vi "list and create PG DI table_1.vi"(8 "error in":errorcluster, 9 "DI table":string[](array[string]), 10 "table name":string, 11 "conn":u32) -> (0 "error out":errorcluster, 3 "conn_out":u32)   [LabVIEW 2019, in "PostgreSQL.lvlib"]
uses:
  PostgreSQL.lvlib
  PostgreSQL2LabVIEW/libpqlv/src/PQresultErrorMessage.vi
  PostgreSQL2LabVIEW/libpqUtility/src/PQclear.vi
  PostgreSQL2LabVIEW/libpqlv/src/PQsendQuery.vi
  PostgreSQL2LabVIEW/libpqlv/src/PQgetResult.vi
  PostgreSQL2LabVIEW/libpqlv/src/PQresultStatus.vi
  PostgreSQL2LabVIEW/libpqUtility/src/PQgetColumn.vi
  PostgreSQL2LabVIEW/libpqlv/src/PQclear.vi
  PostgreSQL2LabVIEW/libpqUtility/src/PQfetchTables.vi
  PostgreSQL2LabVIEW/libpqlv/src/PQgetvalue.vi
  PostgreSQL2LabVIEW/libpqlv/src/PQntuples.vi
  PostgreSQL2LabVIEW/libpqUtility/libpqutility.lvlib
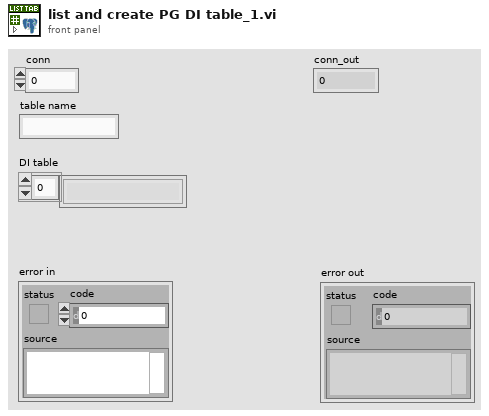
[diagram p1: front panel]
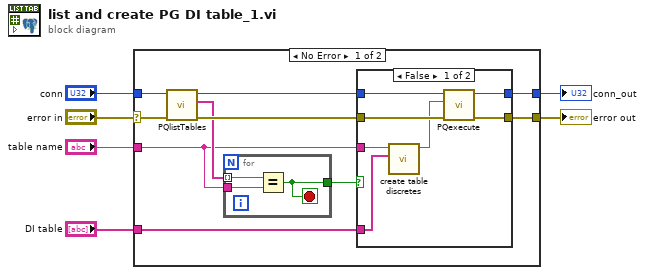
[diagram p0: block diagram]
diagram:
  n1 = case shown="No Error" "error in" {
    selector: "error in" -> [w13 w30]
    tunnel: "conn" -> [w10 w29]
    tunnel: [w16 w29] -> w4
    tunnel: "DI table" -> [w8 _]
    tunnel: [w15 w30] -> w3
    tunnel: "table name" -> [w7 _]
    frame No Error {
      n2 = call "PQlistTables.vi"("error in"=w13, "conn"=w10) -> ("error out"=w12:errorcluster, "Data"=w9:string[], "conn_out"=w11:u32)  [unwired: 7 in]
      n3 = for {
        tunnel: w7 -> [w18]
        tunnel: w9 -> [w19] mode=indexing
        tunnel: [w17] -> w14
        stop <- w17 stop-if-true
        n4 = Equal?(x=w19, y=w18) -> (x = y?=w17:bool)
      }
      n5 = case shown="False" w14 {
        tunnel: w11 -> [w24 w28]
        tunnel: [w21 w28] -> w16
        tunnel: w12 -> [w23 w27]
        tunnel: [w20 w27] -> w15
        tunnel: w8 -> [w25 _]
        tunnel: w7 -> [w26 _]
        frame False {
          n6 = call "create table discretes.vi"("DI table"=w25, "table name"=w26) -> ("create table parameters"=w22:string)  [unwired: 9 in]
          n7 = call "PQexecute.vi"("error in"=w23, "SQL querry"=w22, "conn"=w24) -> ("error out"=w20:errorcluster, "conn_out"=w21:u32)  [unwired: 7 in]
        }
        frame True {
        }
      }
    }
    frame Error {
    }
  }
  "conn_out" <- w4
  "error out" <- w3
